vi "Periodic Tasks.vi"() -> ()   [LabVIEW 2011]
doc: "This VI runs in parallel to other tasks. It can contain as many user-defined periodic loops as you need. These can carry out PID or other sorts of timed response."
uses:
  <vilib>/Platform/TimedLoop/XDataNode/timing_clust.ctl
  <vilib>/Platform/TimedLoop/XDataNode/nitl_modes.ctl
  <vilib>/Platform/TimedLoop/XDataNode/wakeup.ctl
  <vilib>/Rock Robotics/SystemInterfaces/Utilities/FPGA_UtilitiesLED State.ctl
  <vilib>/Rock Robotics/SystemInterfaces/Utilities/FPGA_UtilitiesLED Source.ctl
  <vilib>/Rock Robotics/WPI/Relay/WPI_RelayValue.ctl
  Robot Global Data.vi
  <vilib>/Platform/TimedLoop/XDataNode/XDataNode.xnode
  <vilib>/Platform/TimedLoop/XDataNode/XDNodeRunTimeDep.lvlib
panel:
  in  "Home Speed":dbl
  in  "Home Position":dbl
  out "Current Voltage":dbl
  in  "upper limit":dbl=4.5
  in  "lower limit":dbl=0.85
  # "Speed to move to home"
  # "Target Tracking"
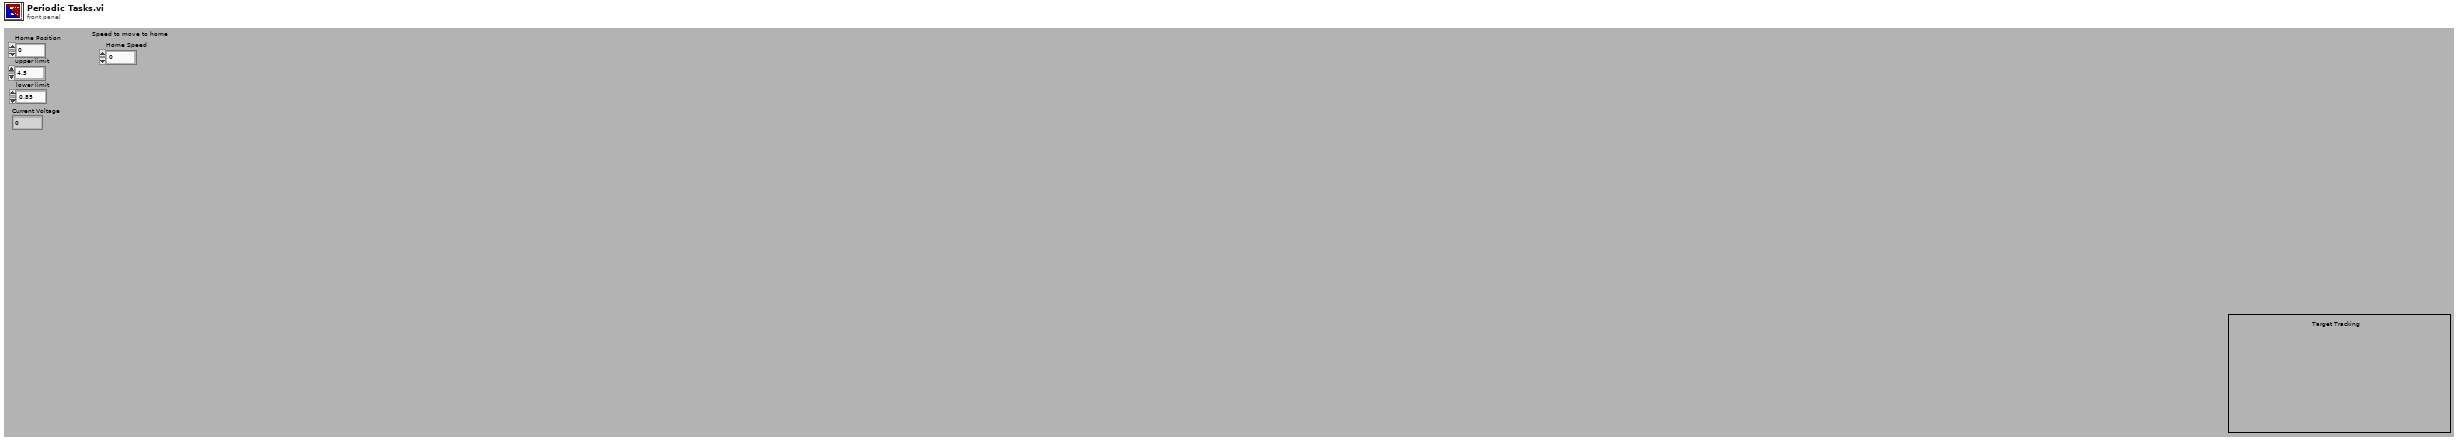
[diagram p1: front panel]
types:
  T1 = typedef "XDNodeRunTimeDep.lvlib/timing_clust.ctl" = cluster{"Expected End [f-1]":u64, "Actual End [f-1]":u64, "Finished Late? [f-1]":bool, "Expected End [i-1]":u64, "Actual End [i-1]":u64, "Finished Late? [i-1]":bool, "Expected Start [i]":u64, "Actual Start [i]":u64, "Expected Start [f]":u64, "Actual Start [f]":u64, "Source Name":string, "Structure Name":string, "Period":i64, "Deadline":i64, "Offset":i64, "Start":i64, "Priority":i32, "Timeout":i32, "Mode":T2, "Wakeup Reason":T3, "Error":errorcluster, "Source Type":string, "Secondary Source Type":string, "Global End Time":u64, "Global Start Time":u64, "Frame Duration":u64, "Iteration Duration":u64, "Assigned CPU":i32, "I/O Scan Engine Mode":u32}
  T2 = typedef "XDNodeRunTimeDep.lvlib/nitl_modes.ctl" = enum32{"No Change", "Process missed periods, maintain original phase", "Discard missed periods, maintain original phase", "Process missed periods, ignore original phase", "Discard missed periods, ignore original phase"}
  T3 = typedef "XDNodeRunTimeDep.lvlib/wakeup.ctl" = enum32{"Normal", "Aborted", "Asynchronous wakeup", "Timing source error", "Timed loop error", "Timeout"}
  T4 = typedef "WPI_RelayValue.ctl" = enum16{"Off", "On", "Forward", "Reverse"}
  T5 = typedef "WPI_AnalogChannelDevRef.ctl" = cluster{"DevStatus":errorcluster, "Analog Module":T6, "Analog Channel":T7}
  T6 = typedef "FPGA_TypedefAnalogModule.ctl" = enum16{"Analog Module 1", "Analog Module 2"}
  T7 = typedef "FPGA_AIChannel.ctl" = enum8{"AI 1", "AI 2", "AI 3", "AI 4", "AI 5", "AI 6", "AI 7", "AI 8", "Invalid"}
  T8 = typedef "WPI_RelayDevRef.ctl" = cluster{"DevStatus":errorcluster, "Relay Channel":T9, "Digital Module":T10, "Relay Direction":T11}
  T9 = typedef "FPGA_DIORelayChannel.ctl" = enum8{"Relay 1", "Relay 2", "Relay 3", "Relay 4", "Relay 5", "Relay 6", "Relay 7", "Relay 8", "Invalid"}
  T10 = typedef "FPGA_TypedefDigitalModule.ctl" = enum16{"Digital Module 1", "Digital Module 2"}
  T11 = typedef "WPI_RelayDirection.ctl" = enum16{"Both directions", "Forward only", "Reverse only"}
  T12 = cluster{"Axis 1":dbl, "Axis 2":dbl, "Axis 3":dbl, "Axis 4":dbl, "Axis 5":dbl, "Axis 6":dbl, "Button 1":bool, "Button 2":bool, "Button 3":bool, "Button 4":bool, "Button 5":bool, "Button 6":bool, "Button 7":bool, "Button 8":bool, "Button 9":bool, "Button 10":bool, "Button 11":bool, "Button 12":bool}
  T13 = cluster{"Driver Station Digital Output (1-8)[0]":bool, "Driver Station Digital Output (1-8)[1]":bool, "Driver Station Digital Output (1-8)[2]":bool, "Driver Station Digital Output (1-8)[3]":bool, "Driver Station Digital Output (1-8)[4]":bool, "Driver Station Digital Output (1-8)[5]":bool, "Driver Station Digital Output (1-8)[6]":bool, "Driver Station Digital Output (1-8)[7]":bool, "Driver Station Digital Output (1-8)[8]":bool}
  T14 = typedef "FPGA_UtilitiesLED State.ctl" = enum16{"Off", "On", "Toggle"}
  T15 = typedef "FPGA_UtilitiesLED Source.ctl" = enum16{"User LED", "FPGA LED"}
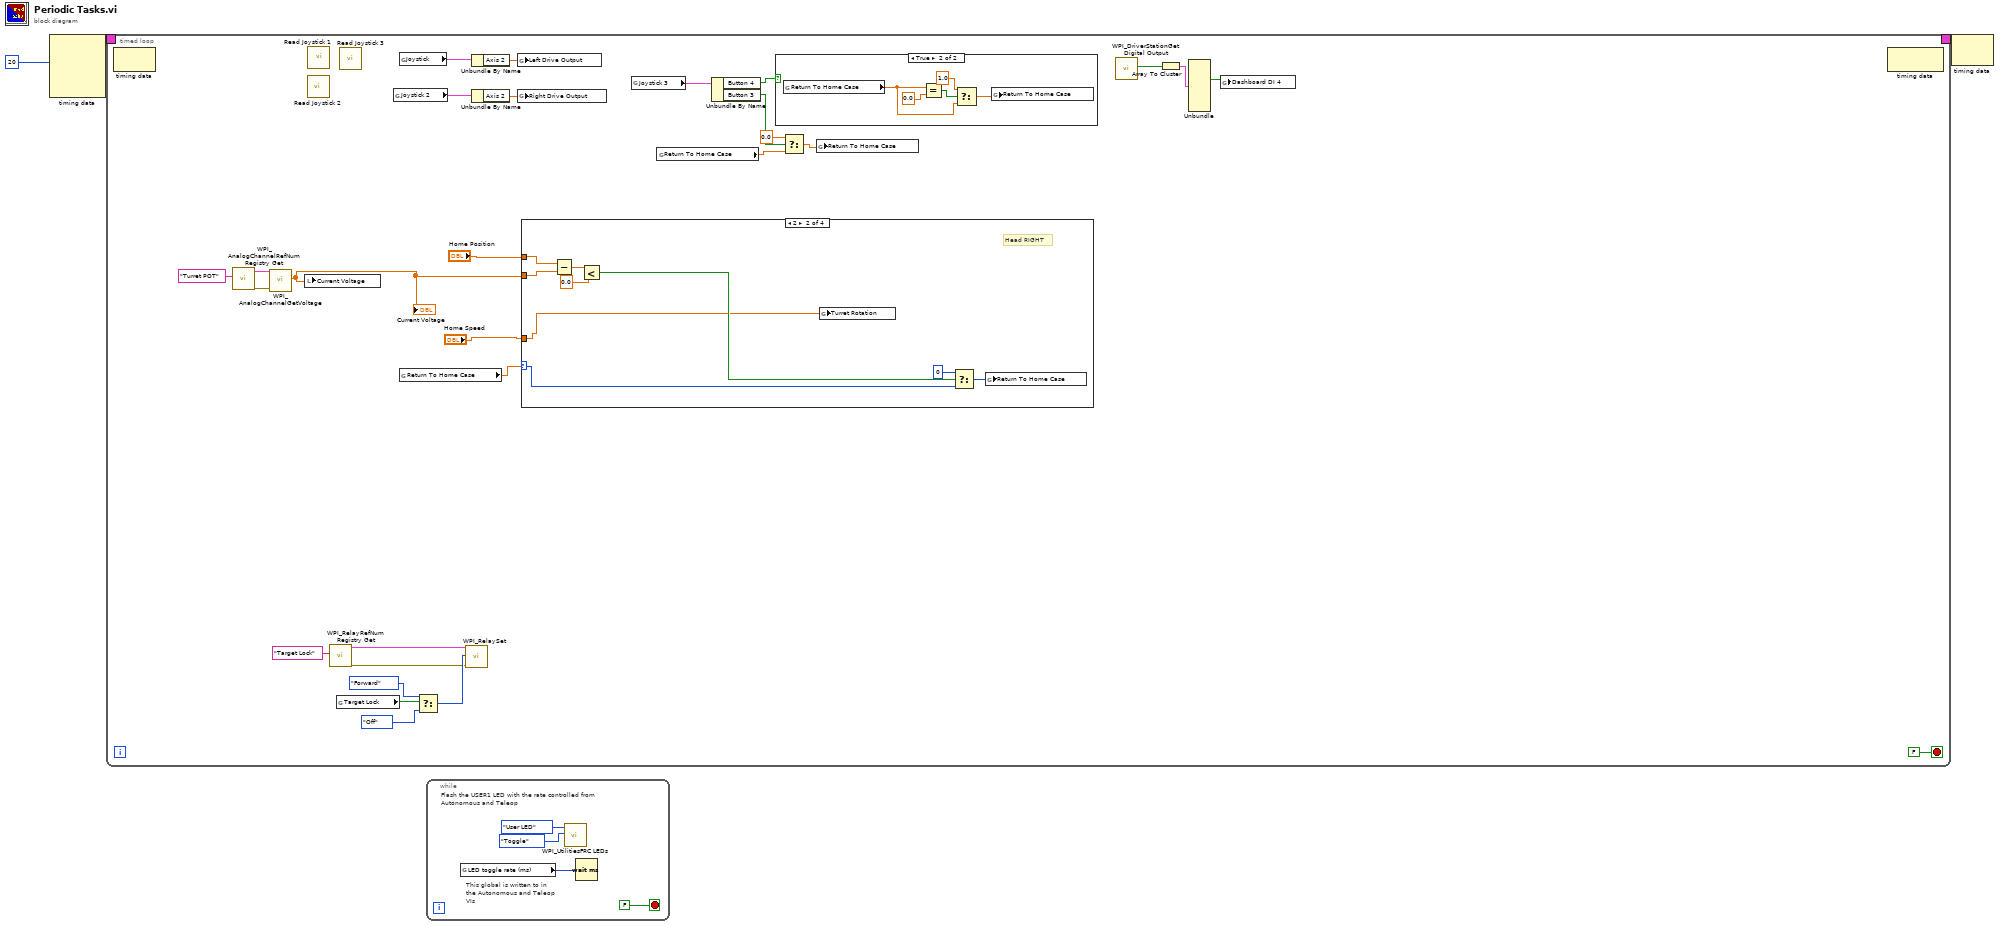
[diagram p0: block diagram]
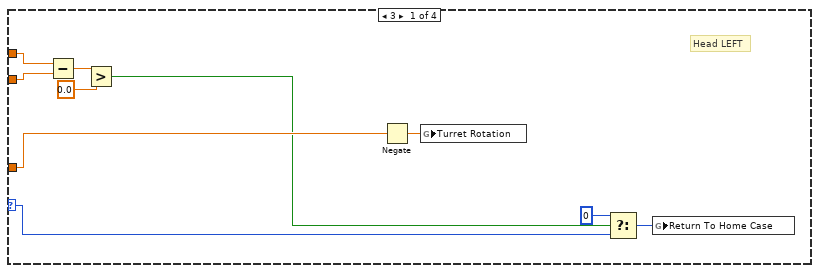
[diagram p2: hidden frame]
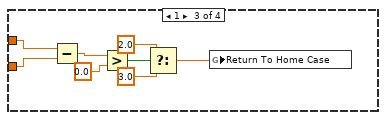
[diagram p3: hidden frame]
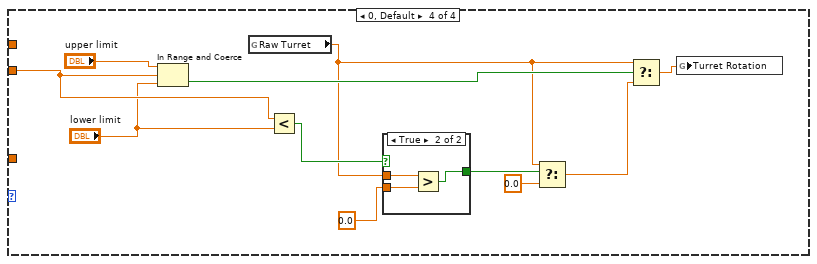
[diagram p4: hidden frame]
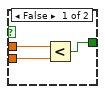
[diagram p5: hidden frame]
diagram:
  n1 = node-c288(i64 20 ("Period")) -> (w3:T1)  [unwired: 3 in]
  n2 = timed-loop {
    timing: w3 -> [_]
    timing-out: [_] -> w2
    stop <- FALSE stop-if-true
    n3 = node-c288() -> ()  [unwired: 1 in, 1 out]
    n4 = call <vilib>:"WPI_AnalogChannelRefNum Registry Get.vi"("refnum name"="Turret POT") -> ("error out"=w14:errorcluster, "AIDeviceRef"=w15:T5)  [unwired: 9 in]
    n5 = call <vilib>:"WPI_AnalogChannelGetVoltage.vi"("error in (no error)"=w14, "AIDeviceRef"=w15) -> ("Voltage"=w11:dbl)  [unwired: 7 in, 2 out]
    "Current Voltage" <- w11
    n6 = local write "Current Voltage"(w11) -> ()
    n7 = call "Read Joystick 2.vi"() -> ()  [unwired: 12 in]
    n8 = call "Read Joystick 1.vi"() -> ()  [unwired: 12 in]
    n9 = call <vilib>:"WPI_RelayRefNum Registry Get.vi"("refnum name"="Target Lock") -> ("error out"=w16:errorcluster, "RelayDevRef"=w17:T8)  [unwired: 9 in]
    n10 = global read "Robot Global Data.vi" "Target Lock"() -> (w22:bool)
    n11 = call "Read Joystick 3.vi"() -> ()  [unwired: 12 in]
    n12 = global read "Robot Global Data.vi" "Joystick 2"() -> (w24:T12)
    n13 = global read "Robot Global Data.vi" "Joystick"() -> (w25:T12)
    n14 = global read "Robot Global Data.vi" "Return To Home Case"() -> (w10:dbl)
    n15 = Select(t=WPI_RelayValue."Forward" ("RelayValue"), s=w22, f=WPI_RelayValue."Off" ("RelayValue")) -> (s? t:f=w19:T4)
    n16 = call <vilib>:"WPI_RelaySet.vi"("error in (no error)"=w16, "RelayValue"=w19, "RelayDevRef"=w17) -> ()  [unwired: 7 in, 2 out]
    n17 = Unbundle By Name(w25) -> ("Axis 2"=w28:dbl)
    n18 = Unbundle By Name(w24) -> ("Axis 2"=w27:dbl)
    n19 = global write "Robot Global Data.vi" "Left Drive Output"(w28) -> ()
    n20 = global write "Robot Global Data.vi" "Right Drive Output"(w27) -> ()
    n21 = case shown="2" w10 {
      selector: w10 -> [w39 w43 _ _]
      tunnel: w11 -> [w35 w44 w57 w69]
      tunnel: "Home Position" -> [w36 w45 w58 _]
      tunnel: "Home Speed" -> [w37 w42 _ _]
      frame 3 {
        # "Head LEFT"
        n22 = Subtract(x=w36, y=w35) -> (x-y=w34:dbl)
        n23 = Greater?(x=w34, y=0.0) -> (0:w32:bool)
        n24 = Negate(x=w37) -> (-x=w38:dbl)
        n25 = global write "Robot Global Data.vi" "Turret Rotation"(w38) -> ()
        n26 = Select(t=0, s=w32, f=w39) -> (s? t:f=w40:i32)
        n27 = global write "Robot Global Data.vi" "Return To Home Case"(w40) -> ()
      }
      frame 2 {
        # "Head RIGHT"
        n28 = Subtract(x=w45, y=w44) -> (x-y=w48:dbl)
        n29 = Less?(x=w48, y=0.0) -> (x < y?=w46:bool)
        n30 = global write "Robot Global Data.vi" "Turret Rotation"(w42) -> ()
        n31 = Select(t=0, s=w46, f=w43) -> (s? t:f=w49:i32)
        n32 = global write "Robot Global Data.vi" "Return To Home Case"(w49) -> ()
      }
      frame 1 {
        n33 = Subtract(x=w58, y=w57) -> (x-y=w56:dbl)
        n34 = Greater?(x=w56, y=0.0) -> (0:w54:bool)
        n35 = Select(t=2.0, s=w54, f=3.0) -> (s? t:f=w51:dbl)
        n36 = global write "Robot Global Data.vi" "Return To Home Case"(w51) -> ()
      }
      frame 0, Default {
        n37 = In Range and Coerce(upper limit="upper limit", x=w69, lower limit="lower limit") -> (In Range?=w66:bool)  [unwired: 1 out]
        n38 = global read "Robot Global Data.vi" "Raw Turret"() -> (w59:dbl)
        n39 = Less?(x=w69, y="lower limit") -> (x < y?=w61:bool)
        n40 = case shown="True" w61 {
          tunnel: 0.0 -> [w71 w75]
          tunnel: [w70 w74] -> w62
          tunnel: w59 -> [w72 w73]
          frame False {
            n41 = Less?(x=w72, y=w71) -> (x < y?=w70:bool)
          }
          frame True {
            n42 = Greater?(x=w73, y=w75) -> (0:w74:bool)
          }
        }
        n43 = Select(t=w59, s=w62, f=0.0) -> (s? t:f=w60:dbl)
        n44 = Select(t=w59, s=w66, f=w60) -> (s? t:f=w68:dbl)
        n45 = global write "Robot Global Data.vi" "Turret Rotation"(w68) -> ()
      }
    }
    n46 = global read "Robot Global Data.vi" "Joystick 3"() -> (w23:T12)
    n47 = global read "Robot Global Data.vi" "Return To Home Case"() -> (w7:dbl)
    n48 = Unbundle By Name(w23) -> ("Button 4"=w26:bool, "Button 3"=w8:bool)
    n49 = case shown="True" w26 {
      frame False {
      }
      frame True {
        n50 = global read "Robot Global Data.vi" "Return To Home Case"() -> (w77:dbl)
        n51 = Equal?(x=w77, y=0.0) -> (x = y?=w79:bool)
        n52 = Select(t=1.0, s=w79, f=w77) -> (s? t:f=w76:dbl)
        n53 = global write "Robot Global Data.vi" "Return To Home Case"(w76) -> ()
      }
    }
    n54 = Select(t=0.0, s=w8, f=w7) -> (s? t:f=w6:dbl)
    n55 = global write "Robot Global Data.vi" "Return To Home Case"(w6) -> ()
    n56 = call <vilib>:"WPI_DriverStationGet Digital Output.vi"() -> ("Driver Station Digital Output (1-8)"=w31:bool[])  [unwired: 10 in, 1 out]
    n57 = Array To Cluster(array=w31) -> (cluster=w30:T13)
    n58 = Unbundle(w30) -> ("Driver Station Digital Output (1-8)[3]"=w29:bool)  [unwired: 8 out]
    n59 = global write "Robot Global Data.vi" "Dashboard DI 4"(w29) -> ()
    n60 = node-c288() -> ()  [unwired: 1 in, 1 out]
  }
  n61 = while {
    stop <- FALSE stop-if-true
    # "This global is written to in the Autonomous and Teleop VIs"
    # "Flash the USER1 LED with the rate controlled from Autonomous and Teleop"
    n62 = global read "Robot Global Data.vi" "LED toggle rate (ms)"() -> (w83:u32)
    n63 = call <vilib>:"WPI_UtilitiesFRC LEDs.vi"("State"=FPGA_UtilitiesLED_State."Toggle", "LED Type"=FPGA_UtilitiesLED_Source."User LED") -> ()  [unwired: 1 in, 9 out]
    n64 = Wait (ms)(milliseconds to wait=w83) -> ()  [unwired: 1 out]
  }
  n65 = node-c288(w2) -> ()  [unwired: 1 out]
